vi "ParseArguments.vi"(8 "error in (no error)":errorcluster, 9 "Inputs":string[](array[string]), 11 "SaveForPrevious in":refnum<class "SaveForPrevious.lvclass">) -> (0 "error out":errorcluster, 3 "SaveForPrevious out":refnum<class "SaveForPrevious.lvclass">)   [LabVIEW 2014, in "SaveForPrevious.lvclass"]
uses:
  SaveForPrevious.lvclass
  <nishared>/LabVIEW CLI/Operations/Utilities/OperationErrorType.ctl
  SaveForPrevious.lvclass/SaveForPrevious.ctl
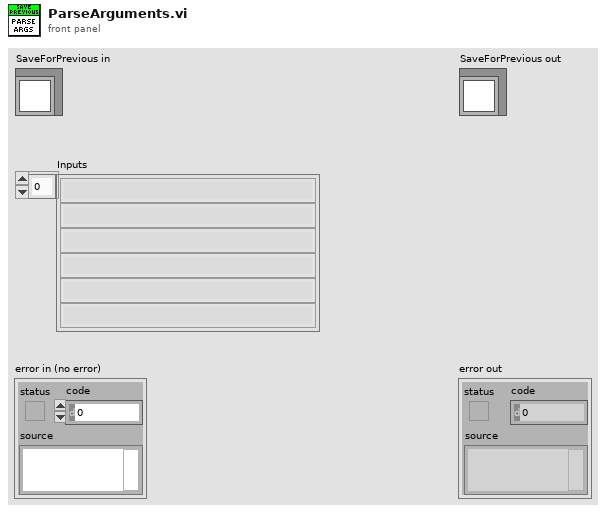
[diagram p1: front panel]
types:
  T1 = typedef "OperationErrorType.ctl" = enum16{"RequiredArgumentMissing", "UnknownArguments", "LoggerSetMultipleTimes", "OperationBrokenError"}
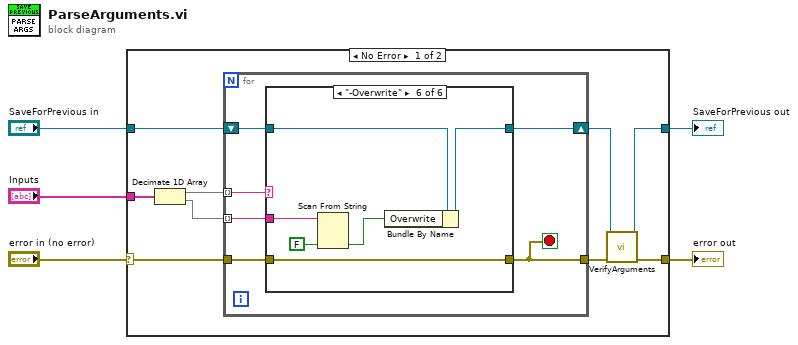
[diagram p0: block diagram]
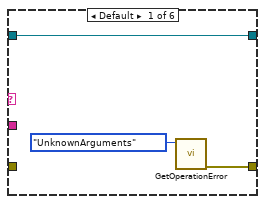
[diagram p2: hidden frame]
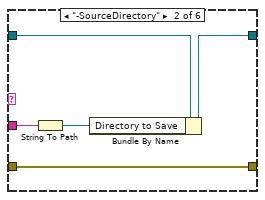
[diagram p3: hidden frame]
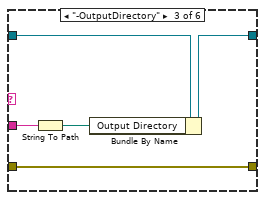
[diagram p4: hidden frame]
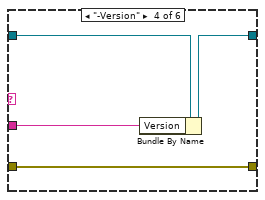
[diagram p5: hidden frame]
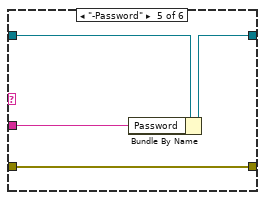
[diagram p6: hidden frame]
diagram:
  n1 = case shown="No Error" "error in (no error)" {
    selector: "error in (no error)" -> [w12 w49]
    tunnel: [w8 w49] -> w4
    tunnel: [w6 w48] -> w2
    tunnel: "SaveForPrevious in" -> [w11 w48]
    tunnel: "Inputs" -> [w10 _]
    frame No Error {
      n2 = Decimate 1D Array(w10) -> (w14:string[], w13:string[])
      n3 = for {
        shift-right: [w19] -> w7
        shift-left: w11 -> [w20]
        tunnel: w14 -> [w18] mode=indexing
        tunnel: w13 -> [w17] mode=indexing
        tunnel: w12 -> [w16]
        tunnel: [w15] -> w9
        stop <- w15 stop-if-true
        n4 = case shown="\"-Overwrite\"" w18 {
          tunnel: w20 -> [w22 w28 w33 w37 w41 w47]
          tunnel: [w22 w26 w31 w35 w39 w46] -> w19
          tunnel: w17 -> [_ w24 w29 w36 w40 w44]
          tunnel: w16 -> [_ w25 w30 w34 w38 w45]
          tunnel: [w21 w25 w30 w34 w38 w45] -> w15
          frame Default {
            n5 = call <nishared>:"GetOperationError.vi"("Operation Error Type"=OperationErrorType."UnknownArguments") -> ("error out"=w21:errorcluster)  [unwired: 10 in]
          }
          frame "-SourceDirectory" {
            n6 = String To Path(string=w24) -> (path=w27:path)
            n7 = Bundle By Name(cluster=w28, "Directory to Save"=w27) -> (w26:refnum<class "SaveForPrevious.lvclass">)
          }
          frame "-OutputDirectory" {
            n8 = String To Path(string=w29) -> (path=w32:path)
            n9 = Bundle By Name(cluster=w33, "Output Directory"=w32) -> (w31:refnum<class "SaveForPrevious.lvclass">)
          }
          frame "-Version" {
            n10 = Bundle By Name(cluster=w37, "Version"=w36) -> (w35:refnum<class "SaveForPrevious.lvclass">)
          }
          frame "-Password" {
            n11 = Bundle By Name(cluster=w41, "Password"=w40) -> (w39:refnum<class "SaveForPrevious.lvclass">)
          }
          frame "-Overwrite" {
            n12 = Scan From String(input string=w44, default 1=FALSE) -> (output 1=w42:bool)  [unwired: 3 in, 3 out]
            n13 = Bundle By Name(cluster=w47, "Overwrite"=w42) -> (w46:refnum<class "SaveForPrevious.lvclass">)
          }
        }
      }
      n14 = call "VerifyArguments.vi"("error in (no error)"=w9, "SaveForPrevious in"=w7) -> ("error out"=w8:errorcluster, "SaveForPrevious out"=w6:refnum<class "SaveForPrevious.lvclass">)  [unwired: 8 in]
    }
    frame Error {
    }
  }
  "error out" <- w4
  "SaveForPrevious out" <- w2
